vi "run.vi"   [LabVIEW 2011]
types:
  T1 = enum32{"Invalid", "Standard", "Closed", "Hidden", "Minimized", "Maximized"}
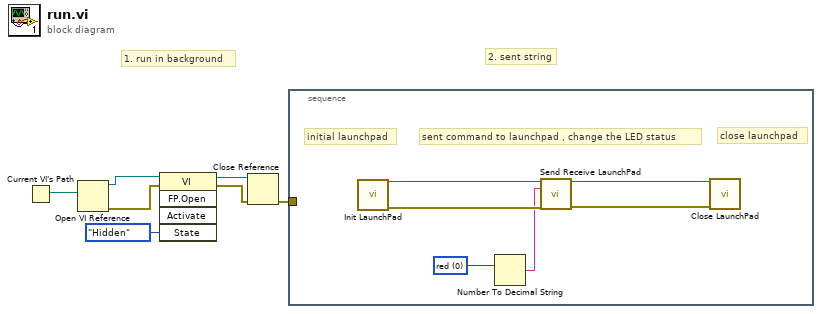
[diagram p0: block diagram]
diagram:
  # "2. sent string"
  # "1. run in background"
  n1 = Current VI's Path() -> (path=w2:path)
  n2 = Open VI Reference(vi path=w2) -> (vi reference=w3:refnum<vi>, error out=w4:errorcluster)  [unwired: 5 in]
  n3 = invoke class="VI" method="FP.Open"(reference=w3, error in=w4, "State"=T1."Hidden") -> (reference out=w6:refnum<vi>, error out=w7:errorcluster)  [unwired: 2 in, 3 out]
  n4 = Close Reference(reference=w6, error in (no error)=w7) -> (error out=w1:errorcluster)
  n5 = stacked-sequence {
    tunnel: w1 -> [_]
    frame #0 {
      w9 = u16 0 items=["red"=0, "green"=6] ("Ring")
      # "close launchpad"
      # "sent command to launchpad , change the LED status"
      # "initial launchpad"
      n6 = call "Init LaunchPad.vi"() -> ("error out"=w10:errorcluster, "VISA resource name out"=w13:refnum<visa-resource-name>)  [unwired: 10 in]
      n7 = Number To Decimal String(number=w9) -> (decimal integer string=w8:string)  [unwired: 1 in]
      n8 = call "Send Receive LaunchPad.vi"("VISA resource"=w13, "write buffer"=w8, "error in"=w10) -> ("VISA resource 2"=w12:refnum<visa-resource-name>, "error out"=w11:errorcluster)  [unwired: 10 in, 1 out]
      n9 = call "Close LaunchPad.vi"("VISA resource name"=w12, "error in"=w11) -> ()  [unwired: 13 in, 1 out]
    }
  }
